vi "PeakFinder.vi"(9 "Trigger location":i32, 10 "Number of Points":dbl, 11 "Input Y values":dbl[](array[numeric])) -> (2 "peak?":bool, 3 "Input Y values":dbl[](array[numeric]))   [LabVIEW 2014]
panel:
  # "Peak Finder VI"
  # "Inputs"
  # "Outputs"
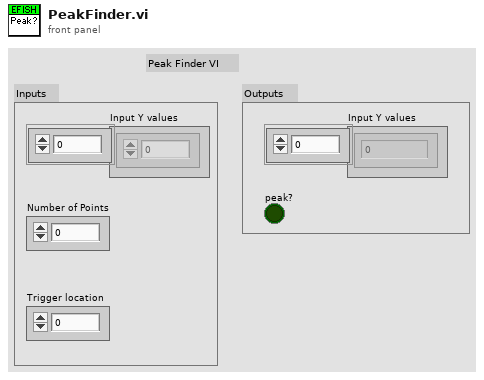
[diagram p1: front panel]
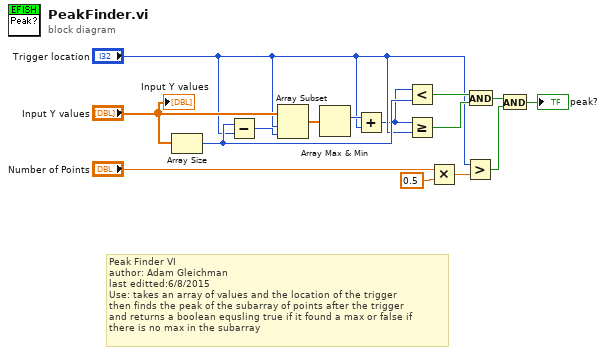
[diagram p0: block diagram]
diagram:
  # "Peak Finder VI\nauthor: Adam Gleichman\nlast editted:6/8/2015\nUse: takes an array of values and the location of the trigger\nthen finds the peak of the subarray of points after the trigger\nand returns a boolean equsling true if it found a max or false if \nthere is no max in the subarray"
  n1 = Array Size(array="Input Y values") -> (size(s)=w9:i32)
  n2 = Subtract(x=w9, y="Trigger location") -> (x-y=w15:i32)
  n3 = Array Subset(array="Input Y values", index="Trigger location", length=w15) -> (w14:dbl[])
  n4 = Array Max & Min(array=w14) -> (max index (indices)=w13:i32)  [unwired: 3 out]
  n5 = Add(x=w13, y="Trigger location") -> (x+y=w1:i32)
  n6 = Less?(x=w1, y=w9) -> (x < y?=w12:bool)
  n7 = Greater Or Equal?(x=w1, y="Trigger location") -> (x >= y?=w11:bool)
  n8 = Multiply(x="Number of Points", y=0.5) -> (x*y=w4:dbl)
  n9 = Greater?(x="Trigger location", y=w4) -> (0:w3:bool)
  n10 = And(x=w12, y=w11) -> (x .and. y?=w8:bool)
  n11 = And(x=w8, y=w3) -> (x .and. y?=→"peak?":bool)
  "Input Y values" <- "Input Y values"
